vi "CRYSet Hardware for Calibrate.vi"() -> (3 "Steps Out":T1[](array[typedef]) {"Repeat State Array"."Start" format="%#_5g"; "Y dB ref" format="%.1f"; "Y data" items=["dB", "Lin"]; "Start" format="%#_5g"})   [LabVIEW 2013]
uses:
  Typedef Control/CRYStep.ctl
  Typedef Control/CRYData Cluster.ctl
  CRYCal Global.vi
  CRYProject/CRYProject Editor Global.vi
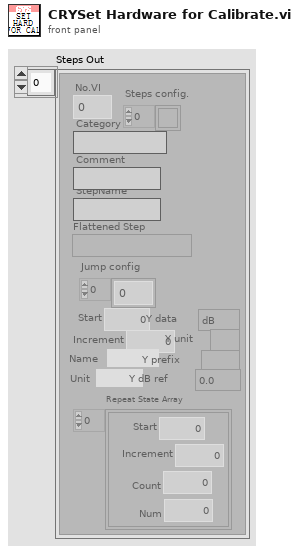
[diagram p1: front panel]
types:
  T1 = typedef "CRYStep.ctl" = cluster{"No.VI":i32, "Category":string, "StepName":string, "Seq setup flattened":string, "Comment":string, "Steps config.":bool[], "Jump config":i32[], "Start":dbl, "Increment":dbl, "Name":string, "Unit":string, "Y data":u16, "Y prefix":string, "Y dB ref":dbl, "Y unit":string, "Repeat State Array":cluster{"Start":dbl, "Increment":dbl, "Count":i32, "Num":i32}[]}
  T2 = typedef "CRYData Cluster.ctl" = cluster{"Name":string, "Curve":cluster{"x":dbl, "y":dbl, "z":dbl}[], "X data":u16, "Y data":u16, "Z data":u16, "X axis":u16, "Y axis":u16, "Z axis":u16, "X unit":string, "Y unit":string, "Z unit":string, "X dB ref":dbl, "Y dB ref":dbl, "Z dB ref":dbl, "single val":bool, "protected":bool, "display X":bool, "display Y":bool, "display Z":bool, "Test Info":string, "Step No.":i32, "Plot Settings":cluster{"Color":u32, "Interpolation":u8, "Point Style":u8, "Line Style":u8, "Point Color":u32, "Line Width":u8, "Bar Plot Style":u8, "Fill To":i16}, "AutoProtect":bool}
  T3 = typedef "CRYTS.ctl" = cluster{"No.TS":u16, "TS File Path":path, "TS Name":string, "EditStepName":string, "Steps":T1[], "New State":bool, "Change State":bool, "Flattened CurveLib Data":string, "Document Data":string, "EditStepNo":u16, "Operator Start File":string, "Sequence Type":string, "Sequence Language":string}
  T4 = typedef "CRYCalibration All Cluster.ctl" = cluster{"Calibration 2D":T5[], "Help":string, "Tab Value":i32, "Input Signal Type":string, "Output Signal Type":string}
  T5 = typedef "CRYCalibration 2DCluster.ctl" = cluster{"Calibration":T6, "Corr Curve":T2, "EQ Curve":T2, "Sens Curve":T2}
  T6 = typedef "CRYCalibration Cluster.ctl" = cluster{"Calibration Step Name":string, "Device":string, "Correction Curve Name":string, "Equalization Curve Name":string, "Sensitivity Curve Name":string, "Corr Folder and File":string, "EQ Folder and File":string, "Sens Folder and File":string, "Corr Step size":u16, "EQ Step size":u16, "Input":bool, "Last Cal Date (sec)":timestamp, "Cha Name":string, "Corr Curve Found":bool, "EQ Curve Found":bool, "Sens Curve Found":bool, "Signal Type":string, "Calibrated Device":string, "Hz":u32}
  T7 = typedef "CRYHardware.ctl" = cluster{"Name":string, "Analog I/O":u16, "Digital I/O":u16, "Channels":u8, "Dig Dev ID":u8, "N ports":u8, "Interface":u32, "Dig I/O Ports":cluster{"port #":i16, "width":i16, "direction":i32}[], "Interf settings":cluster{"Type":u16, "COM Port":u8, "Baud rate":u32, "Data bits":u32, "Parity":u16, "Stop bits":u16, "Flow control":u16, "Dev ID IEEE":u8}[], "N interfs":i32, "udev SNs":i16[], "udev enable":bool, "Channel Array":T8[], "Cal sequence":string, "SelectedIn":u16, "SelectedOut":u16, "SelectedTab":u16, "State":bool, "Help":string, "Advanced":bool, "In Audio Driver":u16, "Out Audio Driver":u16}
  T8 = typedef "CRYHardware Channel Info.ctl" = cluster{"ID":i32, "Name":string, "Digital":bool, "Input":bool, "Device Name":string, "Hardware Ch ID":u8, "Vmax (V)":dbl, "Latency (samples)":dbl, "Sampling Rate (Hz)":u32, "Bit Depth":u32, "Anti-aliasing Factor (%fs)":sgl, "DAQmx Channel":tag, "term config":i32, "Coupling":i32, "IEPE en":bool, "ASIOChannel Name":string, "Audio Driver":u16, "ASIOChannel Index":u8}
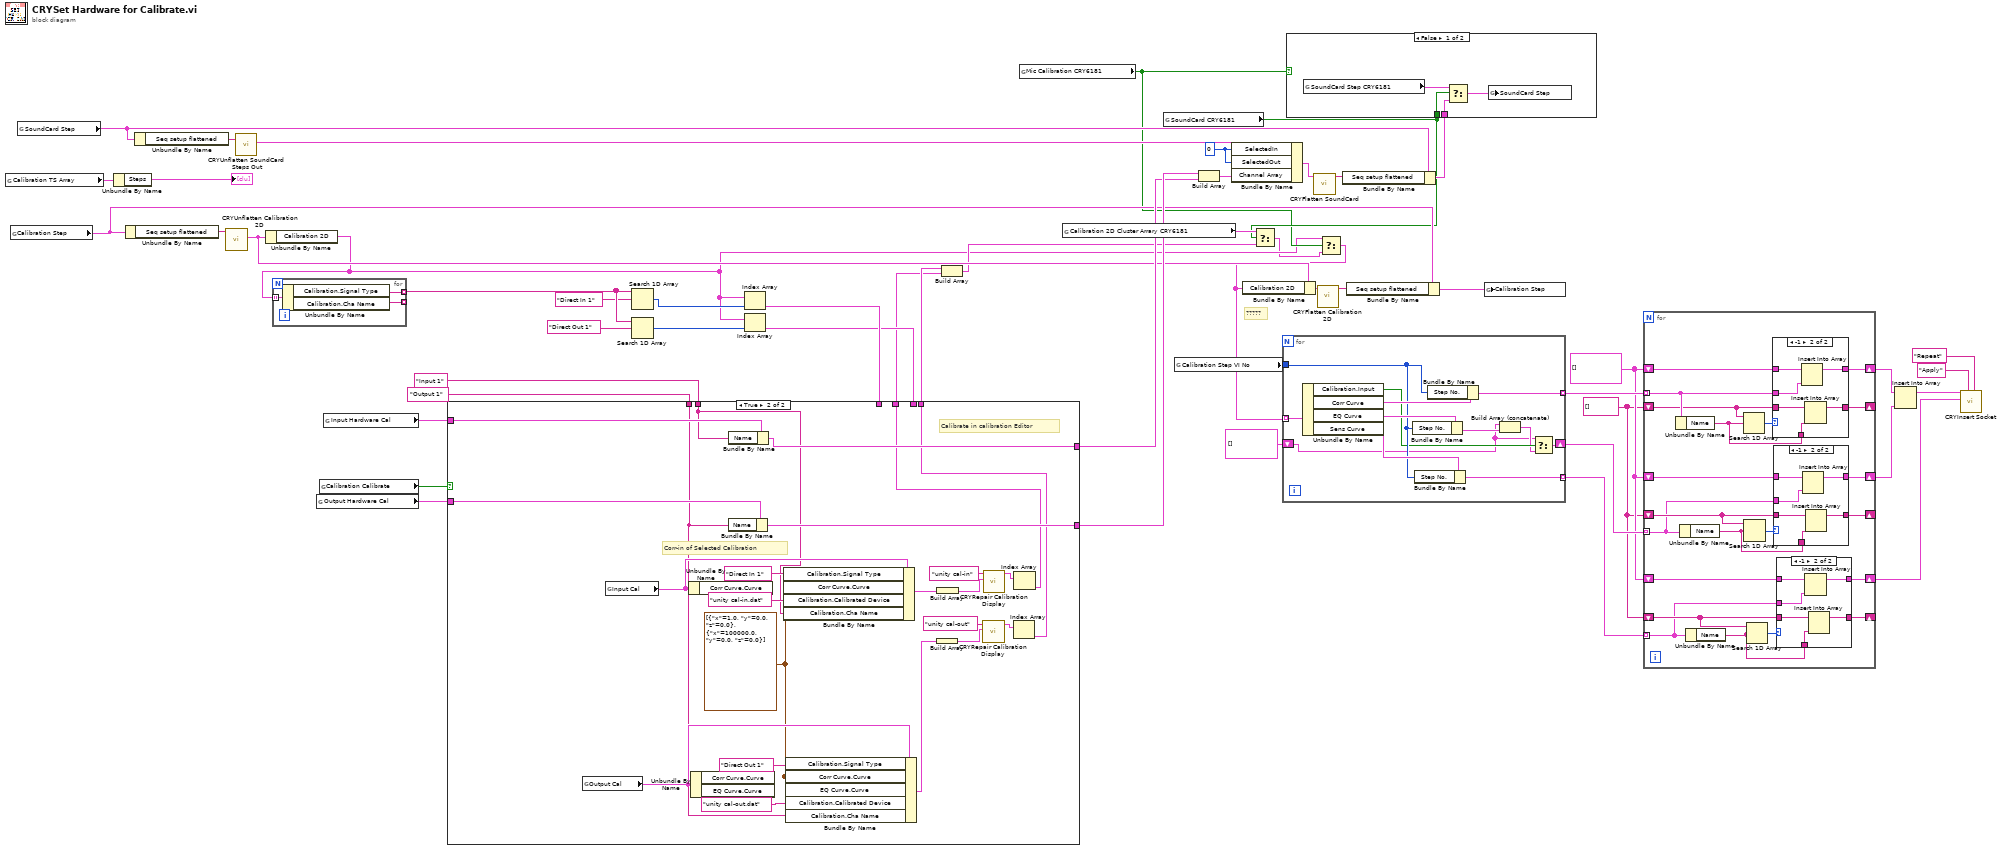
[diagram p0: block diagram]
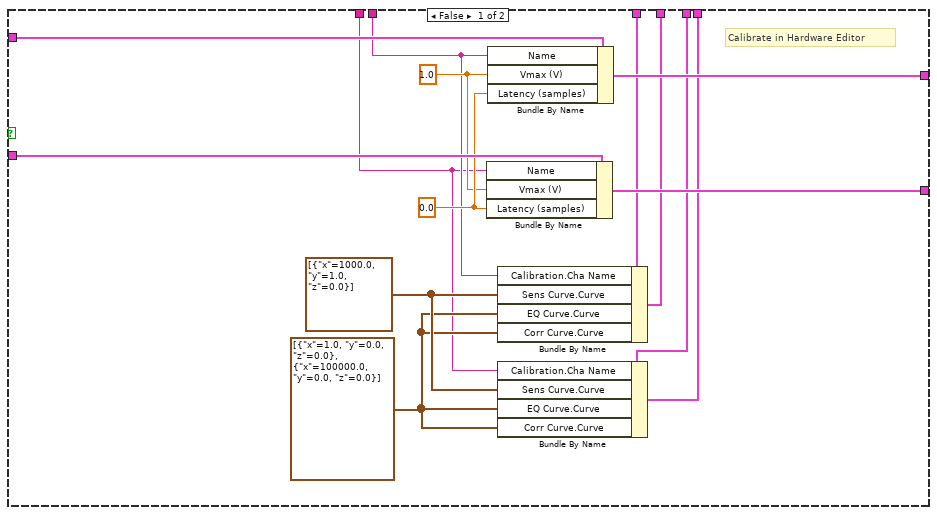
[diagram p6: hidden frame]
diagram:
  w11 = T2[] []
  w10 = string[] []
  w24 = u16 0 ("SelectedIn")
  # "?????"
  n1 = global read "CRYProject Editor Global.vi" "Calibration TS Array"() -> (w26:T3)
  n2 = global read "CRYProject Editor Global.vi" "Calibration Step"() -> (w33:T1)
  n3 = global read "CRYProject Editor Global.vi" "SoundCard Step"() -> (w34:T1)
  n4 = Unbundle By Name(w26) -> ("Steps"=→"Steps Out":T1[])
  n5 = Unbundle By Name(w33) -> ("Seq setup flattened"=w39:string)
  n6 = Unbundle By Name(w34) -> ("Seq setup flattened"=w52:string)
  n7 = call "CRYUnflatten Calibration 2D.vi"("Flattened Calibration"=w39) -> ("Calibration Step Out"=w32:T4)  [unwired: 8 in, 2 out]
  n8 = call "CRYUnflatten SoundCard.vi"("Flatten SoundCard"=w52) -> ("SoundCard"=w18:T7)  [unwired: 8 in, 2 out]
  n9 = Unbundle By Name(w32) -> ("Calibration 2D"=w4:T5[])
  n10 = for {
    tunnel: w4 -> [w55] mode=indexing
    tunnel: [w54] -> w48 mode=indexing
    tunnel: [w53] -> _ mode=indexing
    n11 = Unbundle By Name(w55) -> ("Calibration.Signal Type"=w54:string, "Calibration.Cha Name"=w53:string)
  }
  n12 = global read "CRYCal Global.vi" "Output Hardware Cal"() -> (w47:T8)
  n13 = global read "CRYCal Global.vi" "Calibration Calibrate"() -> (w19:bool)
  n14 = global read "CRYCal Global.vi" "Input Hardware Cal"() -> (w46:T8)
  n15 = Search 1D Array(1D array=w48, element="Direct In 1") -> (index of element=w43:i32)  [unwired: 1 in]
  n16 = Search 1D Array(1D array=w48, element="Direct Out 1") -> (index of element=w42:i32)  [unwired: 1 in]
  n17 = Index Array(array=w4, index=w43) -> (element=w38:T5)
  n18 = Index Array(array=w4, index=w42) -> (element=w37:T5)
  n19 = case shown="True" w19 {
    tunnel: w47 -> [w69 w89]
    tunnel: w46 -> [w68 w91]
    tunnel: "Input 1" -> [w57 w71]
    tunnel: "Output 1" -> [w56 w70]
    tunnel: [w67 w90] -> w45
    tunnel: [w66 w92] -> w44
    tunnel: w38 -> [w63 _]
    tunnel: w37 -> [w61 _]
    tunnel: [w60 w72] -> w36
    tunnel: [w62 w74] -> w35
    frame False {
      w58 = cluster{"x":dbl, "y":dbl, "z":dbl}[] [{"x"=1.0, "y"=0.0, "z"=0.0}, {"x"=100000.0, "y"=0.0, "z"=0.0}] ("EQ Curve.Curve")
      w59 = cluster{"x":dbl, "y":dbl, "z":dbl}[] [{"x"=1000.0, "y"=1.0, "z"=0.0}] ("Sens Curve.Curve")
      w65 = 0.0 ("Vmax (V)")
      w64 = 1.0 ("Vmax (V)")
      # "Calibrate in Hardware Editor"
      n20 = Bundle By Name(cluster=w69, "Name"=w56, "Vmax (V)"=w64, "Latency (samples)"=w65) -> (w67:T8)
      n21 = Bundle By Name(cluster=w68, "Name"=w57, "Vmax (V)"=w64, "Latency (samples)"=w65) -> (w66:T8)
      n22 = Bundle By Name(cluster=w63, "Calibration.Cha Name"=w57, "Sens Curve.Curve"=w59, "EQ Curve.Curve"=w58, "Corr Curve.Curve"=w58) -> (w62:T5)
      n23 = Bundle By Name(cluster=w61, "Calibration.Cha Name"=w56, "Sens Curve.Curve"=w59, "EQ Curve.Curve"=w58, "Corr Curve.Curve"=w58) -> (w60:T5)
    }
    frame True {
      w83 = cluster{"x":dbl, "y":dbl, "z":dbl}[] [{"x"=1.0, "y"=0.0, "z"=0.0}, {"x"=100000.0, "y"=0.0, "z"=0.0}] ("EQ Curve.Curve")
      # "Calibrate in calibration Editor"
      # "Corr-in of Selected Calibration"
      n24 = global read "CRYCal Global.vi" "Output Cal"() -> (w86:T5)
      n25 = global read "CRYCal Global.vi" "Input Cal"() -> (w88:T5)
      n26 = Unbundle By Name(w88) -> ()  [unwired: 1 out]
      n27 = Unbundle By Name(w86) -> ()  [unwired: 2 out]
      n28 = Bundle By Name(cluster=w89, "Name"=w70) -> (w90:T8)
      n29 = Bundle By Name(cluster=w91, "Name"=w71) -> (w92:T8)
      n30 = Bundle By Name(cluster=w88, "Calibration.Signal Type"="Direct In 1", "Corr Curve.Curve"=w83, "Calibration.Calibrated Device"="unity cal-in.dat", "Calibration.Cha Name"=w71) -> (w77:T5)
      n31 = Bundle By Name(cluster=w86, "Calibration.Signal Type"="Direct Out 1", "Corr Curve.Curve"=w83, "EQ Curve.Curve"=w83, "Calibration.Calibrated Device"="unity cal-out.dat", "Calibration.Cha Name"=w70) -> (w81:T5)
      n32 = Build Array(w81) -> (w80:T5[])
      n33 = Build Array(w77) -> (w79:T5[])
      n34 = call "CRYRepair Calibration Display.vi"("Calibration In"=w80, "Calibration Step Name"="unity cal-out") -> ("Calibration Out"=w73:T5[])  [unwired: 1 in, 8 out]
      n35 = call "CRYRepair Calibration Display.vi"("Calibration In"=w79, "Calibration Step Name"="unity cal-in") -> ("Calibration Out"=w75:T5[])  [unwired: 1 in, 8 out]
      n36 = Index Array(array=w73) -> (element=w72:T5)  [unwired: 1 in]
      n37 = Index Array(array=w75) -> (element=w74:T5)  [unwired: 1 in]
    }
  }
  n38 = Build Array(w36, w35) -> (w15:T5[])
  n39 = global read "CRYCal Global.vi" "Mic Calibration CRY6181"() -> (w5:bool)
  n40 = global read "CRYCal Global.vi" "Calibration 2D Cluster Arrary CRY6181"() -> (w16:T5[])
  n41 = global read "CRYCal Global.vi" "SoundCard CRY6181"() -> (w6:bool)
  n42 = global read "CRYProject Editor Global.vi" "Calibration Step VI No"() -> (w31:i32)
  n43 = Build Array(w45, w44) -> (w50:T8[])
  n44 = Bundle By Name(cluster=w18, "SelectedIn"=w24, "SelectedOut"=w24, "Channel Array"=w50) -> (w49:T7)
  n45 = Select(t=w16, s=w6, f=w15) -> (s? t:f=w3:T5[])
  n46 = call "CRYFlatten SoundCard.vi"("SoundCard"=w49) -> ("SoundCard flattened"=w51:string)  [unwired: 10 in]
  n47 = Select(t=w4, s=w5, f=w3) -> (s? t:f=w2:T5[])
  n48 = Bundle By Name(cluster=w32, "Calibration 2D"=w2) -> (w41:T4)
  n49 = for {
    tunnel: w2 -> [w104] mode=indexing
    tunnel: w31 -> [w100]
    tunnel: [w99] -> w12 mode=indexing
    tunnel: [w98] -> w14 mode=indexing
    shift-right: [w96] -> w13
    shift-left: T2[] [] ("output array") -> [w93]
    n50 = Unbundle By Name(w104) -> ("Calibration.Input"=w97:bool, "Corr Curve"=w103:T2, "EQ Curve"=w102:T2, "Sens Curve"=w101:T2)
    n51 = Bundle By Name(cluster=w102, "Step No."=w100) -> (w95:T2)
    n52 = Bundle By Name(cluster=w101, "Step No."=w100) -> (w99:T2)
    n53 = Bundle By Name(cluster=w103, "Step No."=w100) -> (w98:T2)
    n54 = Build Array (concatenate)(w93, w95) -> (w94:T2[])
    n55 = Select(t=w93, s=w97, f=w94) -> (s? t:f=w96:T2[])
  }
  n56 = call "CRYFlatten Calibration 2D.vi"("Calibration All Cluster"=w41) -> ("Calibration flattened"=w40:string)  [unwired: 10 in]
  n57 = Bundle By Name(cluster=w34, "Seq setup flattened"=w51) -> (w17:T1)
  n58 = case shown="False" w5 {
    tunnel: w17 -> [w107 _]
    tunnel: w6 -> [w105 _]
    frame False {
      n59 = global read "CRYCal Global.vi" "SoundCard Step CRY6181"() -> (w108:T1)
      n60 = Select(t=w108, s=w105, f=w107) -> (s? t:f=w106:T1)
      n61 = global write "CRYProject Editor Global.vi" "SoundCard Step"(w106) -> ()
    }
    frame True {
    }
  }
  n62 = Bundle By Name(cluster=w33, "Seq setup flattened"=w40) -> (w1:T1)
  n63 = global write "CRYProject Editor Global.vi" "Calibration Step"(w1) -> ()
  n64 = for {
    tunnel: w14 -> [w126] mode=indexing
    tunnel: w13 -> [w114] mode=indexing
    tunnel: w12 -> [w115] mode=indexing
    shift-right: [w124] -> _
    shift-left: w10 -> [w125]
    shift-right: [w127] -> w9
    shift-left: w11 -> [w128]
    shift-right: [w120] -> w8
    shift-left: w11 -> [w121]
    shift-right: [w113] -> w7
    shift-left: w11 -> [w119]
    shift-right: [w117] -> _
    shift-left: w10 -> [w118]
    shift-right: [w112] -> _
    shift-left: w10 -> [w116]
    n65 = Unbundle By Name(w126) -> ("Name"=w111:string)
    n66 = Unbundle By Name(w114) -> ("Name"=w110:string)
    n67 = Unbundle By Name(w115) -> ("Name"=w109:string)
    n68 = Search 1D Array(1D array=w125, element=w111) -> (index of element=w129:i32)  [unwired: 1 in]
    n69 = Search 1D Array(1D array=w118, element=w110) -> (index of element=w123:i32)  [unwired: 1 in]
    n70 = Search 1D Array(1D array=w116, element=w109) -> (index of element=w122:i32)  [unwired: 1 in]
    n71 = case shown="-1" w129 {
      tunnel: w128 -> [w147 w153]
      tunnel: [w147 w152] -> w127
      tunnel: w126 -> [_ w151]
      tunnel: w125 -> [w146 w150]
      tunnel: [w146 w149] -> w124
      tunnel: w111 -> [_ w148]
      frame 0, Default {
      }
      frame -1 {
        n72 = Insert Into Array(array=w153, new element=w151) -> (w152:T2[])  [unwired: 1 in]
        n73 = Insert Into Array(array=w150, new element=w148) -> (w149:string[])  [unwired: 1 in]
      }
    }
    n74 = case shown="-1" w123 {
      tunnel: w121 -> [w139 w145]
      tunnel: [w139 w144] -> w120
      tunnel: w114 -> [_ w143]
      tunnel: w118 -> [w138 w142]
      tunnel: [w138 w141] -> w117
      tunnel: w110 -> [_ w140]
      frame 0, Default {
      }
      frame -1 {
        n75 = Insert Into Array(array=w145, new element=w143) -> (w144:T2[])  [unwired: 1 in]
        n76 = Insert Into Array(array=w142, new element=w140) -> (w141:string[])  [unwired: 1 in]
      }
    }
    n77 = case shown="-1" w122 {
      tunnel: w119 -> [w131 w137]
      tunnel: [w131 w136] -> w113
      tunnel: w115 -> [_ w135]
      tunnel: w116 -> [w130 w134]
      tunnel: [w130 w133] -> w112
      tunnel: w109 -> [_ w132]
      frame 0, Default {
      }
      frame -1 {
        n78 = Insert Into Array(array=w137, new element=w135) -> (w136:T2[])  [unwired: 1 in]
        n79 = Insert Into Array(array=w134, new element=w132) -> (w133:string[])  [unwired: 1 in]
      }
    }
  }
  n80 = Insert Into Array(array=w9, new element=w8) -> (w30:T2[])  [unwired: 1 in]
  n81 = call "CRYInsert Socket.vi"("sOption2"="Repeat", "sOption1"="Apply", "Values"=w7, "Curves"=w30) -> ()  [unwired: 7 in, 1 out]
